vi "kernel32_GetVolumeInformationA.vi"(0 "RootPathName(c:\\)":string="c:\\", 11 "error in (no error)":errorcluster caption="错误输入（无错误）") -> (4 "dup RootPathName":string="c:\\", 6 "FileSystemFlags":u32, 8 "FileSystemName":string, 10 "VolumeSerialNumber":u32, 15 "error out":errorcluster caption="错误输出")   [LabVIEW 2011]
uses:
  kernel32.dll
panel:
  out "VolumeName":string
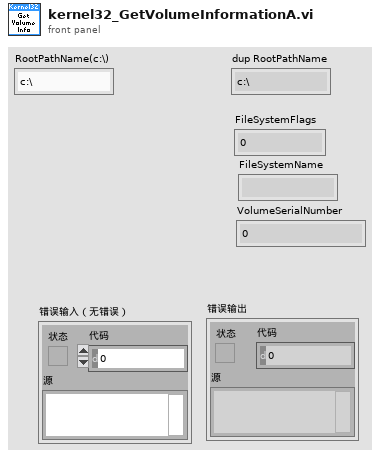
[diagram p1: front panel]
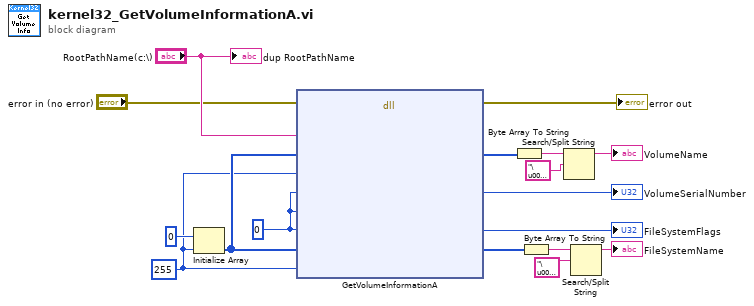
[diagram p0: block diagram]
diagram:
  w14 = u32 255 ("nVolumeNameSize")
  w17 = u32 0 ("lpRootPathName")
  n1 = Initialize Array(u8 0, w14) -> (w16:u8[])
  n2 = dll-call lib="kernel32.dll" fn="GetVolumeInformationA" ("Get VolumeInformation")(error in="error in (no error)", "lpRootPathName"="RootPathName(c:\\)", "lpVolumeNameBuffer"=w16, "nVolumeNameSize"=w14, "lpVolumeSerialNumber"=w17, "lpMaximumComponentLength"=w17, "lpFileSystemFlags"=w17, "lpFileSystemNameBuffer"=w16, "nFileSystemNameSize"=w14) -> (error out=→"error out":errorcluster, "lpVolumeNameBuffer"=w12:u8[], "lpVolumeSerialNumber"=→"VolumeSerialNumber":u32, "lpFileSystemFlags"=→"FileSystemFlags":u32, "lpFileSystemNameBuffer"=w5:u8[])  [unwired: 5 in, 3 out]
  n3 = Byte Array To String(unsigned byte array=w12) -> (string=w10:string)
  n4 = Byte Array To String(unsigned byte array=w5) -> (string=w6:string)
  n5 = Search/Split String(string=w10, search string/char (-)="\u0000" ("search char (-)")) -> (substring before match=→"VolumeName":string)  [unwired: 3 out]
  n6 = Search/Split String(string=w6, search string/char (-)="\u0000" ("search char (-)")) -> (substring before match=→"FileSystemName":string)  [unwired: 3 out]
  "dup RootPathName" <- "RootPathName(c:\\)"
